vi "Disp all.vi"(1 "Temp":dbl, 2 "Time":string="%", 3 "milliseconds to wait betweeen frames":u32, 4 "VISA resource name":refnum<visa-resource-name>, 5 "Temp Colour":u32(colorbox), 6 "Intensity 0-100":dbl(knob) min=0.0 max=100.0 step=1.0 scale=0.0..100.0, 7 "Hum":dbl, 8 "Date":string, 9 "Hum Colour":u32(colorbox)) -> (0 "VISA resource name 2":refnum<visa-resource-name>)   [LabVIEW 2021]
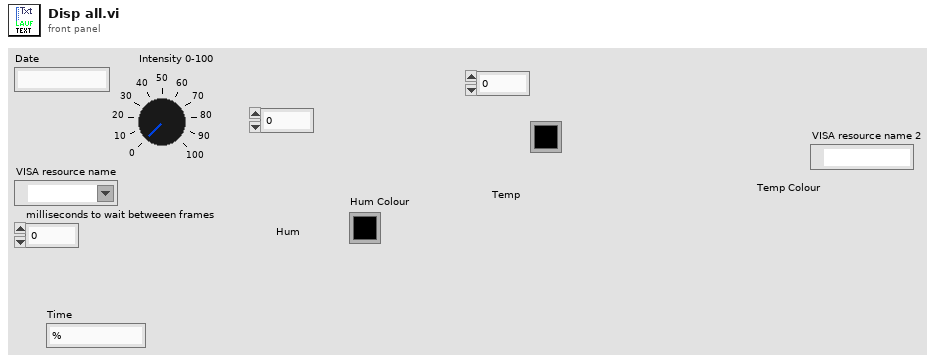
[diagram p1: front panel]
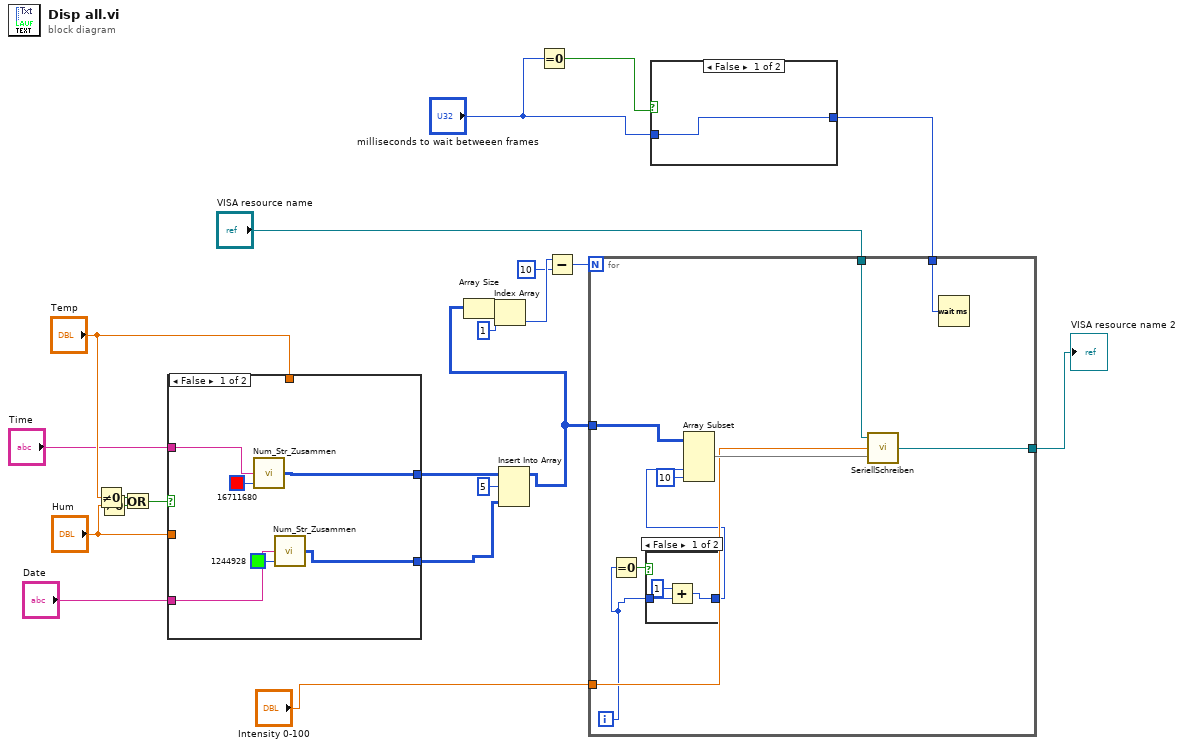
[diagram p0: block diagram]
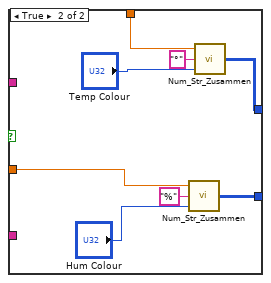
[diagram p2: hidden frame]
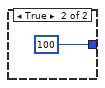
[diagram p3: hidden frame]
diagram:
  n1 = Not Equal To 0?(x="Temp") -> (x != 0?=w6:bool)
  n2 = Not Equal To 0?(x="Hum") -> (x != 0?=w5:bool)
  n3 = Or(x=w6, y=w5) -> (x .or. y?=w7:bool)
  n4 = case shown="False" w7 {
    tunnel: "Temp" -> [_ w36]
    tunnel: "Hum" -> [_ w33]
    tunnel: [w28 w30] -> w20
    tunnel: [w26 w29] -> w19
    tunnel: "Time" -> [w27 _]
    tunnel: "Date" -> [w25 _]
    frame False {
      n5 = call "Num_Str_Zusammen.vi"("Color Box"=u32 16711680, "string"=w27) -> ("Array"=w28:u32[][])  [unwired: 1 in]
      n6 = call "Num_Str_Zusammen.vi"("Color Box"=u32 1244928, "string"=w25) -> ("Array"=w26:u32[][])  [unwired: 1 in]
    }
    frame True {
      n7 = call "Num_Str_Zusammen.vi"("Color Box"="Hum Colour", "string"="%", "number"=w33) -> ("Array"=w29:u32[][])
      n8 = call "Num_Str_Zusammen.vi"("Color Box"="Temp Colour", "string"="°", "number"=w36) -> ("Array"=w30:u32[][])
    }
  }
  n9 = Insert Into Array(array=w20, index (row)=5, new element=w19) -> (w17:u32[][])  [unwired: 1 in]
  n10 = Array Size(array=w17) -> (size(s)=w22:i32[])
  n11 = Index Array(array=w22, index=1) -> (element=w9:i32)
  n12 = Equal To 0?(x="milliseconds to wait betweeen frames") -> (x = 0?=w12:bool)
  n13 = Subtract(x=w9, y=10) -> (x-y=w10:i32)
  n14 = case shown="False" w12 {
    tunnel: "milliseconds to wait betweeen frames" -> [w37 _]
    tunnel: [w37 u32 100 ("milliseconds to wait")] -> w11
    frame False {
    }
    frame True {
    }
  }
  n15 = for {
    N: w10 -> [_]
    tunnel: w17 -> [w48]
    tunnel: "VISA resource name" -> [w45]
    tunnel: [w44] -> w16
    tunnel: "Intensity 0-100" -> [w43]
    tunnel: w11 -> [w42]
    i -> [w39]
    n16 = Equal To 0?(x=w39) -> (x = 0?=w40:bool)
    n17 = case shown="False" w40 {
      tunnel: [w51 w52] -> w41
      tunnel: w39 -> [w50 w52]
      frame False {
        n18 = Add(x=1, y=w50) -> (x+y=w51:i32)
      }
      frame True {
      }
    }
    n19 = Array Subset(array=w48, index (col)=w41, length (col)=10 ("length")) -> (w46:u32[][])  [unwired: 2 in]
    n20 = call "SeriellSchreiben.vi"("Array 100*100 rgb"=w46, "Intensity 0-100"=w43, "VISA resource name"=w45) -> ("VISA resource name 2"=w44:refnum<visa-resource-name>)
    n21 = Wait (ms)(milliseconds to wait=w42) -> ()  [unwired: 1 out]
  }
  "VISA resource name 2" <- w16
